vi "Sort Array of Clusters 2012 NIVerified.vi"(11 "Unsorted Array":T1(array[cluster])) -> (3 "Sorted Array":T1(array[cluster]))   [LabVIEW 2018, in "Support Library.lvlib"]
doc: "This VI sorts an array of clusters by one of its cluster elements. Run the VI. Then select the element you want to sort by from the \"Element to Sort by\" listbox."
uses:
  Support Library.lvlib
panel:
  # "Overview: This VI sorts an array of clusters by one of its cluster elements.\nRequirements: LabVIEW 2012 (or compatible)\nInstructions:\n1. Run the VI\n2. Select an entry from the \"Element to Sort by\" control\n3. Note that the output array is now sorted based on your selection"
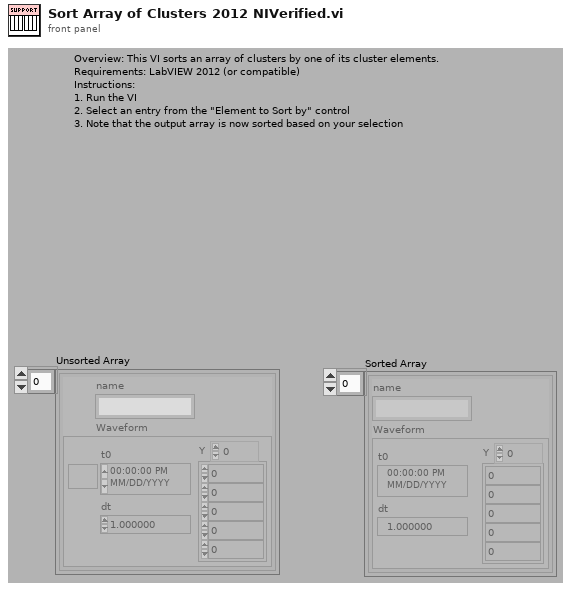
[diagram p1: front panel]
types:
  T1 = cluster{"name":string, "Waveform":waveform(dbl)}[]
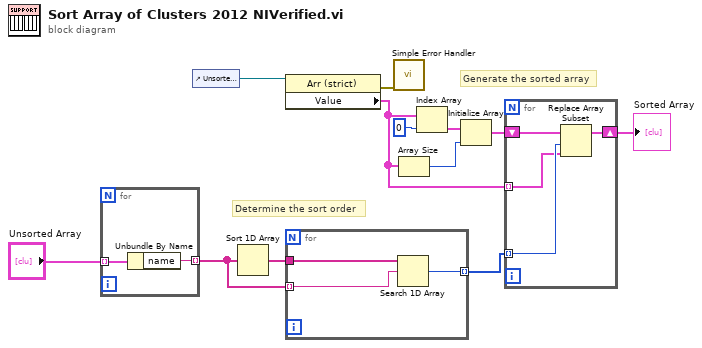
[diagram p0: block diagram]
diagram:
  # "Generate the sorted array"
  # "Determine the sort order"
  n1 = for {
    tunnel: [w14] -> w6 mode=indexing
    tunnel: "Unsorted Array" -> [w13] mode=indexing
    n2 = Unbundle By Name(w13) -> ("name"=w14:string)
  }
  n3 = control-ref of="Unsorted Array"() -> (w3:refnum<vi>)
  n4 = Sort 1D Array(array=w6) -> (sorted array=w1:string[])
  n5 = property class="Arr (strict)"(reference=w3) -> (error out=w5:errorcluster, "Value"=w8:T1)  [unwired: 1 in, 1 out]
  n6 = for {
    tunnel: w6 -> [w16] mode=indexing
    tunnel: w1 -> [w17]
    tunnel: [w15] -> w7 mode=indexing
    n7 = Search 1D Array(1D array=w17, element=w16) -> (index of element=w15:i32)  [unwired: 1 in]
  }
  n8 = call <vilib>:"Simple Error Handler.vi"("error in (no error)"=w5) -> ()  [unwired: 4 in, 5 out]
  n9 = Array Size(array=w8) -> (size(s)=w12:i32)
  n10 = Index Array(array=w8, index=0) -> (element=w10:cluster{"name":string, "Waveform":waveform(dbl)})
  n11 = Initialize Array(w10, w12) -> (w9:T1)
  n12 = for {
    tunnel: w7 -> [w19] mode=indexing
    shift-right: [w20] -> w2
    shift-left: w9 -> [w21]
    tunnel: w8 -> [w18] mode=indexing
    n13 = Replace Array Subset(array=w21, new element=w18, index=w19) -> (w20:T1)
  }
  "Sorted Array" <- w2
